vi "Main.vi"() -> ()   [LabVIEW 2021]
uses:
  Controls/Base_Station_Emulator.ctl
  Controls/Cellular_Technology.ctl
  Enum.ctl
  Controls/TCP_FGV.ctl
panel:
  in  "PPCH NB":string(combo)="6"
  in  "UL fre":i64=-95000000
  in  "DL fre":u64=2655000000
  in  "Eutra Bands 4G":string(combo)="3"
  in  "Add_subscriber":T1={"value"="11111111111111111111111111111111", "Add_Subscriber"="//add_subscriber", "N"=1, "imsi"="10.2.0.1", "phone_no"=0, "key_value"="8baf473f2f8fd09487cccbd7097c6862", "op/opc_value"="opc", "mnc-length"=""} {"phone_no" min=0 max=2; "N" min=1 max=2}
  in  "Hardware input":T2(ring)
  in  "Tab":enum32{"2G", "4G", "5G"}(tab)
  in  "cell":T3(ring)
  in  "Phy":T4(ring)
  in  "gprs":T5(ring)
  in  "Config2G":enum16{"Hardware", "cell", "phy", "gprs"}(ring)
  in  "UL POWER":i32=-13
  in  "dl power":i32=-13
  in  "CELL":T6(ring)
  in  "PHY":T7(ring)
  in  "RRC":T8(ring)
  in  "Config4G":enum16{"hardware", "cell", "phy", "rrc"}(ring)
  in  "dl power 2":i32=-13
  in  "UL POWER 2":i32=-13
  in  "Delete_Subscriber":string="//Delete_subscriber"
  in  "Set sim Config":bool
  in  "Cellular Technology":T9
  in  "Base Station":T10
  in  "Enter":bool
  in  "Stop":bool
  in  "stop emulator":bool
  in  "Start":bool
  out "error out":errorcluster
  in  "error in (no error)":errorcluster
  # "2655000000"
  # "-95000000"
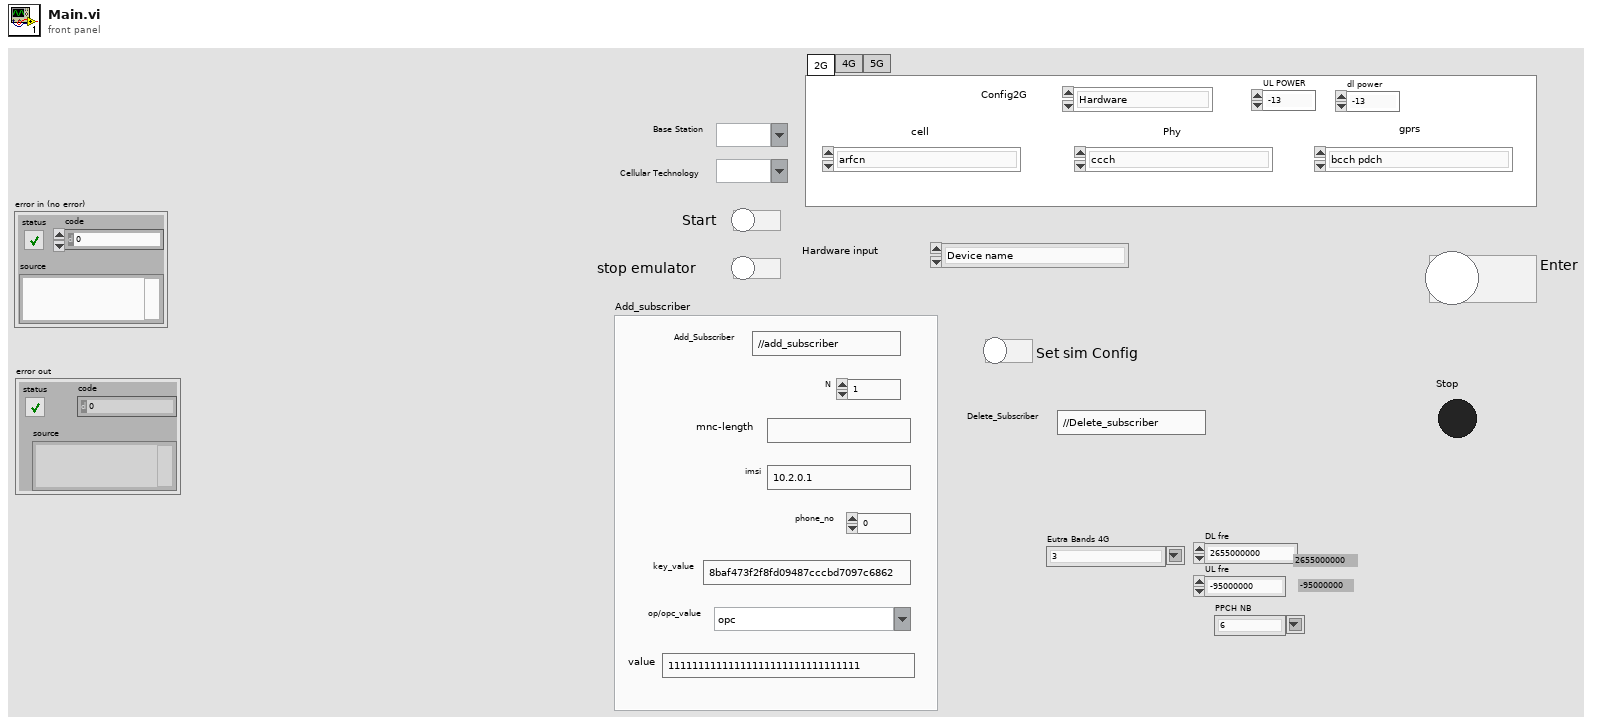
[diagram p1: front panel]
types:
  T1 = cluster{"value":string, "Add_Subscriber":string, "N":i32, "imsi":string, "phone_no":i32, "key_value":string, "op/opc_value":string, "mnc-length":string}
  T2 = enum16{"Device name", "serial name", "dl power", "dl antenna", "ul ref power", "ul antenna"}
  T3 = enum16{"arfcn", "call enables", "cell barred access", "early classmark sending", "fre format", "gprs enabled", "location aea code", "loop back enabled", "mcc", "mnc", "power offset", "si type", "sms enabled"}
  T4 = enum16{"ccch", "add reselect", "attach detach", "block for acs", "cell reselect", "dtx", "hal rate", "min received sig", "multiframe forpg", "pow con indi", "pow contro level", "Rach access control access", "rach call", "RAch maxi retranmission", "rach transmission slots", "radio link timout", "t3212"}
  T5 = enum16{"bcch pdch", "gprs parameter alpha", "access burst", "nack countdown", "network control", "priority access", "rac", "t3168", "t3192"}
  T6 = enum16{"Carrier BW", "DL Frequency", "Duplex Mode", "Eutra operating band", "Measurement report", "MNC length", "MCC", "MNC", "network name", "Physical Cell ID", "Tracking area code", "Transmission Mode", "UL frequency"}
  T7 = enum16{"BCCH modi Coeff", "pbch Repetition", "pcch Narrowband", "pcch pg cycle", "pdsch power boost", "pdsch Ref power", "phich duration", "phish resource", "prach config index", "prach contention resolution", "prach initial received target", "prach maximum transmission", "prach ramping step size", "prach response window", "prach root sequence", "pussh an occassions", "pucch cqi num of RB", "pucch cs antenna", "pucch delta shift", "pucch harq max", "pucch power offset", "pusch alpha", "pusch dmrs enable", "pusch power offset", "srs enable"}
  T8 = enum16{"rlc maxi retransmission", "rlc poll byte", "rlc poll pdu", "rlc timer poll retransmit", "rlc timer reordering", "rlc timer status prohibit"}
  T9 = typedef "Cellular_Technology.ctl" = string
  T10 = typedef "Base_Station_Emulator.ctl" = string
  T11 = typedef "Enum.ctl" = enum16{"Init", "poll", "Start", "Stop", "Config", "Set sim", "Config-4G", "Config-5G"}
  T12 = typedef "TCP_FGV.ctl" = enum16{"Open", "Read", "Write", "Close"}
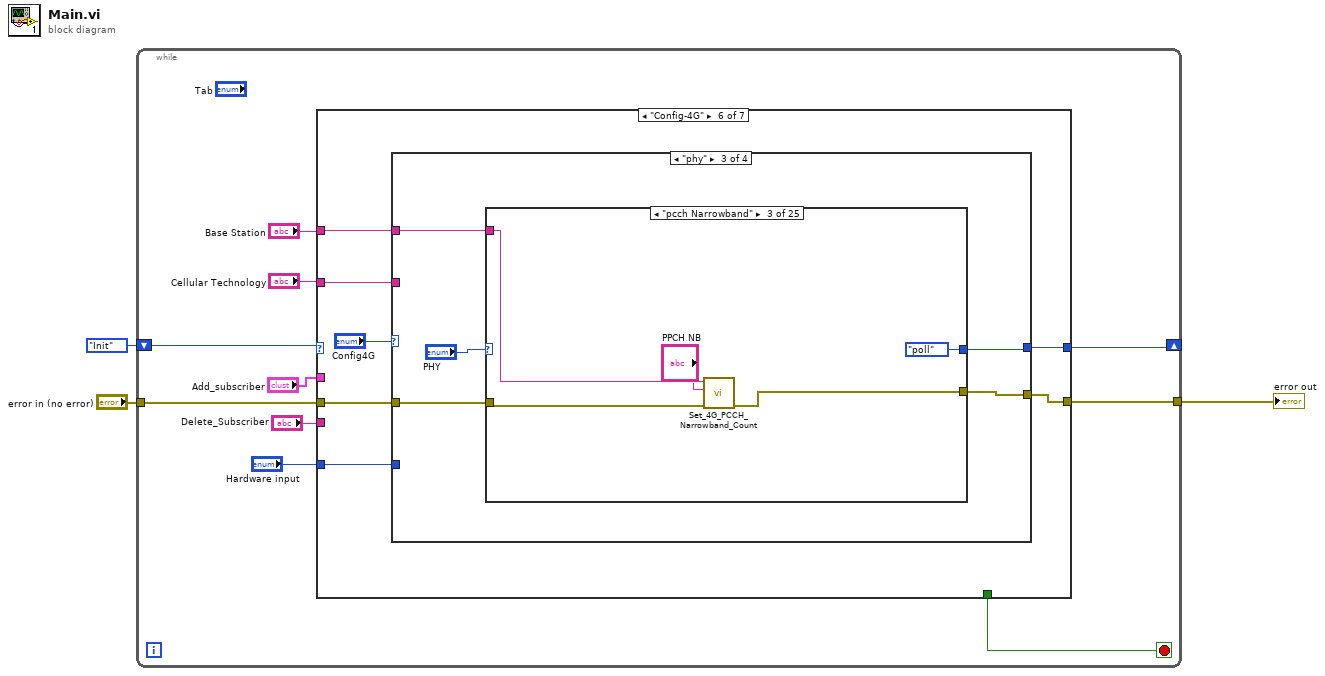
[diagram p0: block diagram]
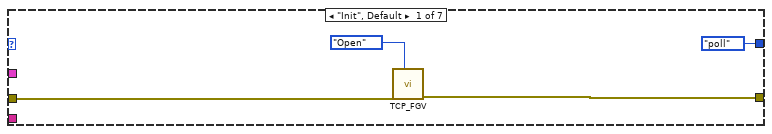
[diagram p2: hidden frame]
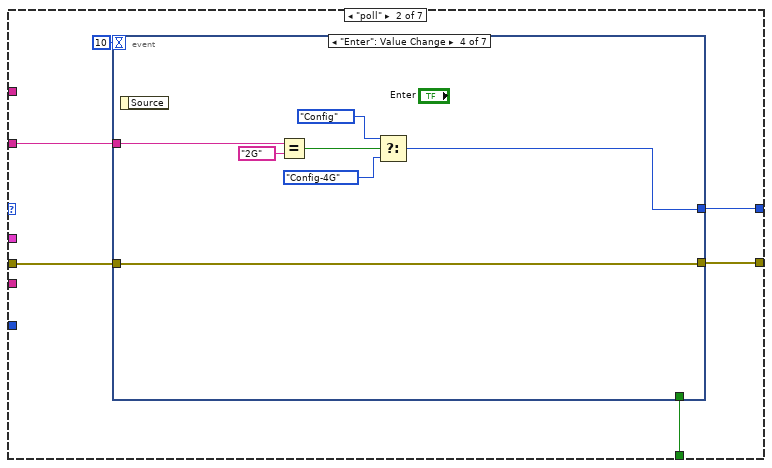
[diagram p3: hidden frame]
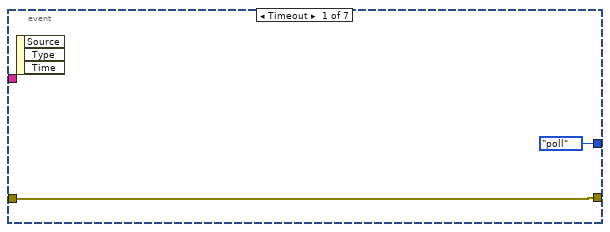
[diagram p4: hidden frame]
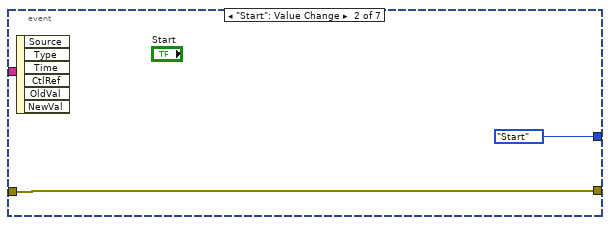
[diagram p5: hidden frame]
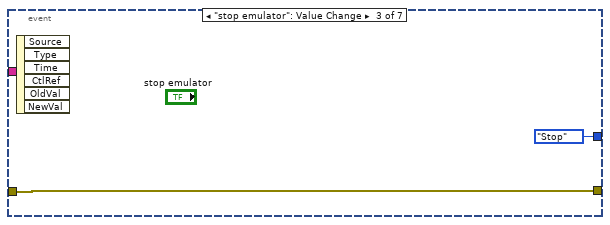
[diagram p6: hidden frame]
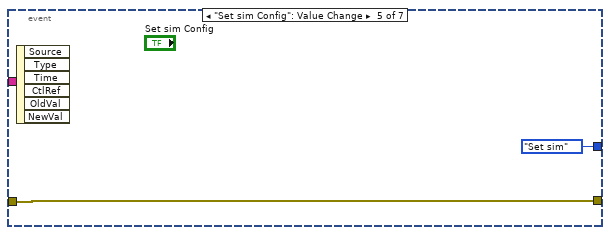
[diagram p7: hidden frame]
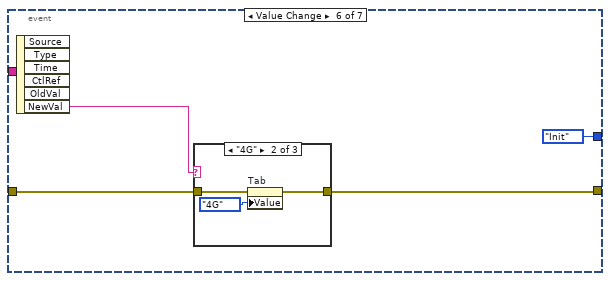
[diagram p8: hidden frame]
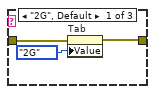
[diagram p9: hidden frame]
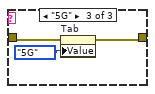
[diagram p10: hidden frame]
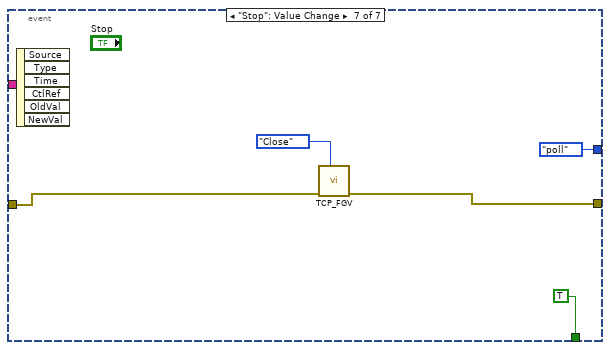
[diagram p11: hidden frame]
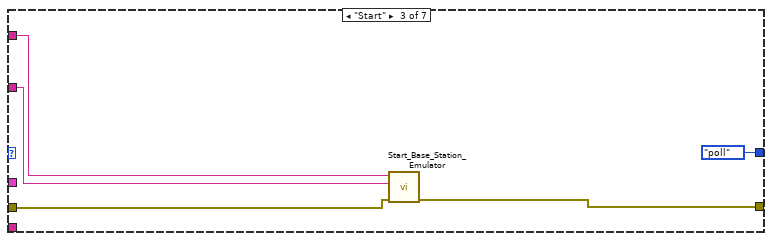
[diagram p12: hidden frame]
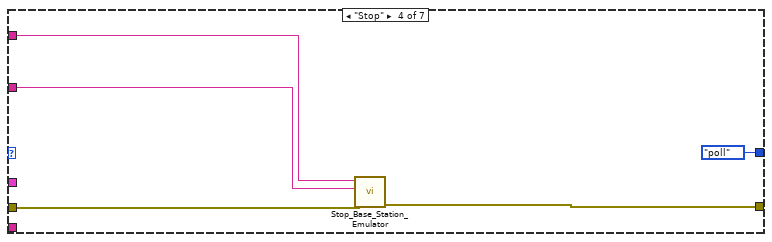
[diagram p13: hidden frame]
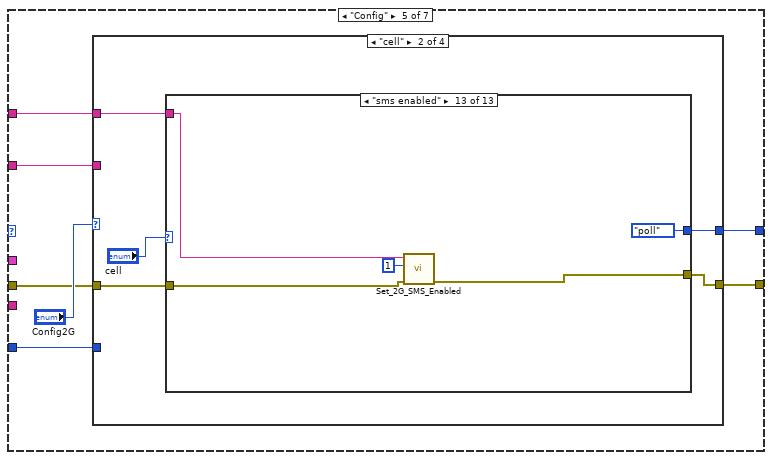
[diagram p14: hidden frame]
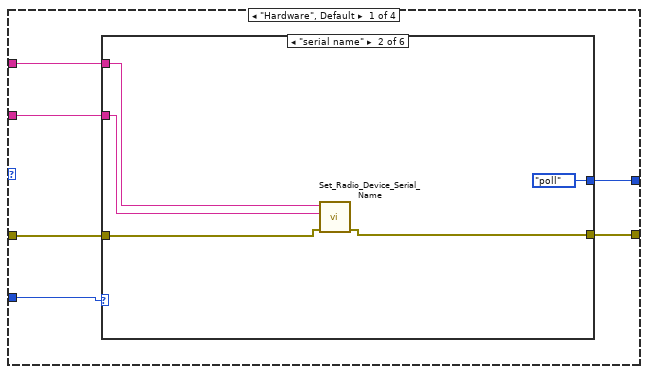
[diagram p15: hidden frame]
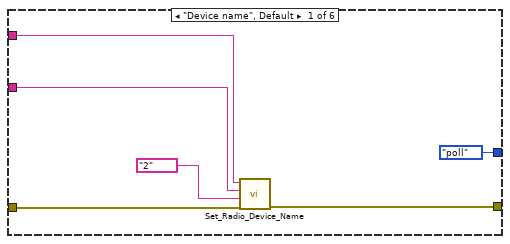
[diagram p16: hidden frame]
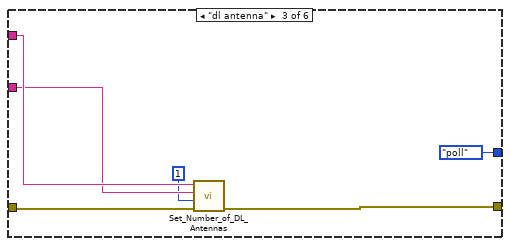
[diagram p17: hidden frame]
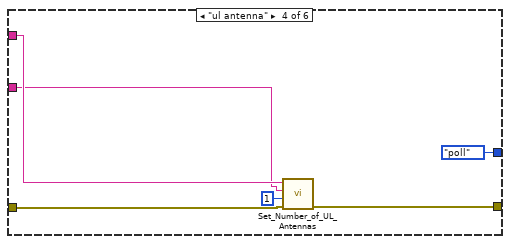
[diagram p18: hidden frame]
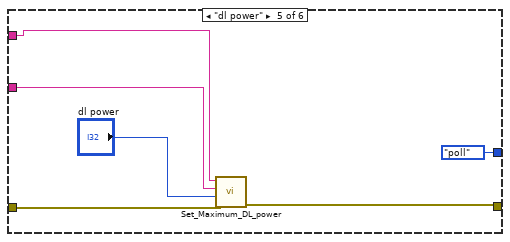
[diagram p19: hidden frame]
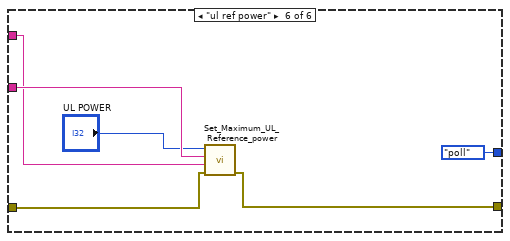
[diagram p20: hidden frame]
diagram:
  n1 = while {
    shift-right: [w12] -> _
    shift-left: Enum."Init" -> [w13]
    tunnel: "error in (no error)" -> [w11]
    tunnel: [w10] -> w1
    stop <- w9 stop-if-true
    n2 = case shown="\"Config-4G\"" w13 {
      tunnel: [Enum."poll" w22 Enum."poll" Enum."poll" w68 w326 w604] -> w12
      tunnel: w11 -> [w16 w21 w61 w66 w72 w330 w608]
      tunnel: [w15 w20 w60 w65 w69 w327 w607] -> w10
      tunnel: "Base Station" -> [_ _ w58 w63 w71 w329 _]
      tunnel: "Cellular Technology" -> [_ w18 w57 w62 w70 w328 _]
      tunnel: "Delete_Subscriber" -> [_ _ _ _ _ _ w606]
      tunnel: [_ w19 _ _ _ _ _] -> w9
      tunnel: "Add_subscriber" -> [_ _ _ _ _ _ w605]
      tunnel: "Hardware input" -> [_ _ _ _ w67 w325 _]
      frame "Init", Default {
        n3 = call "TCP_FGV.vi"("error in (no error)"=w16, "Operation"=TCP_FGV."Open") -> ("error out"=w15:errorcluster)  [unwired: 7 in, 1 out]
      }
      frame "poll" {
        n4 = event shown="[3] \"Enter\": Value Change" {
          selector: _ -> [_ _ _ _ _ _ _]
          dyn-events: _ -> [_ _ _ _ _ _ _]
          timeout: 10 -> [_ _ _ _ _ _ _]
          tunnel: [Enum."poll" Enum."Start" Enum."Stop" w31 Enum."Set sim" Enum."Init" Enum."poll"] -> w22
          tunnel: w21 -> [w24 w26 w28 w36 w38 w41 w54]
          tunnel: [w24 w26 w28 w36 w38 w42 w53] -> w20
          tunnel: [_ _ _ _ _ _ TRUE] -> w19
          tunnel: w18 -> [_ _ _ w35 _ _ _]
          event Timeout {
            n5 = event-data() -> ()  [unwired: 1 in, 3 out]
          }
          event "Start": Value Change {
            n6 = event-data() -> ()  [unwired: 1 in, 6 out]
          }
          event "stop emulator": Value Change {
            n7 = event-data() -> ()  [unwired: 1 in, 6 out]
          }
          event "Enter": Value Change {
            n8 = event-data() -> ()  [unwired: 1 in, 1 out]
            n9 = Equal?(x=w35, y=T9 "2G") -> (x = y?=w33:bool)
            n10 = Select(t=Enum."Config", s=w33, f=Enum."Config-4G") -> (s? t:f=w31:T11)
          }
          event "Set sim Config": Value Change {
            n11 = event-data() -> ()  [unwired: 1 in, 6 out]
          }
          event Value Change {
            n12 = event-data() -> ("NewVal"=w40:T9)  [unwired: 1 in, 5 out]
            n13 = case shown="\"4G\"" w40 {
              tunnel: [w44 w48 w51] -> w42
              tunnel: w41 -> [w45 w47 w50]
              frame "2G", Default {
                n14 = property on="Tab" class="TabCtl (strict)"(error in=w45, "Value"=enum32{"2G", "4G", "5G"}."2G" ("Tab")) -> (error out=w44:errorcluster)  [unwired: 1 in, 1 out]
              }
              frame "4G" {
                n15 = property on="Tab" class="TabCtl (strict)"(error in=w47, "Value"=enum32{"2G", "4G", "5G"}."4G" ("Tab")) -> (error out=w48:errorcluster)  [unwired: 1 in, 1 out]
              }
              frame "5G" {
                n16 = property on="Tab" class="TabCtl (strict)"(error in=w50, "Value"=enum32{"2G", "4G", "5G"}."5G" ("Tab")) -> (error out=w51:errorcluster)  [unwired: 1 in, 1 out]
              }
            }
          }
          event "Stop": Value Change {
            n17 = event-data() -> ()  [unwired: 1 in, 6 out]
            n18 = call "TCP_FGV.vi"("error in (no error)"=w54, "Operation"=TCP_FGV."Close") -> ("error out"=w53:errorcluster)  [unwired: 7 in, 1 out]
          }
        }
      }
      frame "Start" {
        n19 = call "Start_Base_Station_Emulator.vi"("error in (no error)"=w61, "Cellular Technology"=w57, "Base Station"=w58) -> ("error out"=w60:errorcluster)  [unwired: 7 in, 1 out]
      }
      frame "Stop" {
        n20 = call "Stop_Base_Station_Emulator.vi"("error in (no error)"=w66, "Cellular Technology"=w62, "Base Station"=w63) -> ("error out"=w65:errorcluster)  [unwired: 7 in, 1 out]
      }
      frame "Config" {
        n21 = case shown="\"cell\"" "Config2G" {
          tunnel: w72 -> [w79 w117 w188 w277]
          tunnel: w71 -> [w78 w116 w185 w275]
          tunnel: w70 -> [w77 _ _ _]
          tunnel: [w76 w115 w187 w276] -> w69
          tunnel: [w75 w118 w186 w279] -> w68
          tunnel: w67 -> [w74 _ _ _]
          frame "Hardware", Default {
            n22 = case shown="\"serial name\"" w74 {
              tunnel: w79 -> [w85 w90 w94 w102 w108 w112]
              tunnel: [w84 w89 w93 w101 w107 w111] -> w76
              tunnel: w78 -> [w83 w88 w96 w100 w105 w113]
              tunnel: w77 -> [w82 w87 w95 w99 w104 w114]
              tunnel: [Enum."poll" Enum."poll" Enum."poll" Enum."poll" Enum."poll" Enum."poll"] -> w75
              frame "Device name", Default {
                n23 = call "Set_Radio_Device_Name.vi"("error in (no error)"=w85, "value"="2", "Cellular Technology"=w82, "Base Station"=w83) -> ("error out"=w84:errorcluster)  [unwired: 6 in, 1 out]
              }
              frame "serial name" {
                n24 = call "Set_Radio_Device_Serial_Name.vi"("error in (no error)"=w90, "Cellular Technology"=w87, "Base Station"=w88) -> ("error out"=w89:errorcluster)  [unwired: 7 in, 1 out]
              }
              frame "dl antenna" {
                n25 = call "Set_Number_of_DL_Antennas.vi"("error in (no error)"=w94, "No of DL antennas Value"=1, "Cellular Technology"=w95, "Base Station"=w96) -> ("error out"=w93:errorcluster)  [unwired: 6 in, 1 out]
              }
              frame "ul antenna" {
                n26 = call "Set_Number_of_UL_Antennas.vi"("error in (no error)"=w102, "No of UL antennas Value"=1, "Cellular Technology"=w99, "Base Station"=w100) -> ("error out"=w101:errorcluster)  [unwired: 6 in, 1 out]
              }
              frame "dl power" {
                n27 = call "Set_Maximum_DL_power.vi"("error in (no error)"=w108, "No of DL antennas Value"="dl power", "Cellular Technology"=w104, "Base Station"=w105) -> ("error out"=w107:errorcluster)  [unwired: 6 in, 1 out]
              }
              frame "ul ref power" {
                n28 = call "Set_Maximum_UL_Reference_power.vi"("error in (no error)"=w112, "Base Station"=w113, "Cellular Technology"=w114, "No of DL antennas Value"="UL POWER") -> ("error out"=w111:errorcluster)  [unwired: 6 in, 1 out]
              }
            }
          }
          frame "cell" {
            n29 = case shown="\"sms enabled\"" "cell" {
              tunnel: [Enum."poll" Enum."poll" Enum."poll" Enum."poll" Enum."poll" Enum."poll" Enum."poll" Enum."poll" Enum."poll" Enum."poll" Enum."poll" Enum."poll" Enum."poll"] -> w118
              tunnel: w117 -> [w123 w129 w134 w138 w144 w149 w154 w158 w164 w169 w174 w179 w184]
              tunnel: w116 -> [w122 w127 w131 w136 w142 w147 w151 w156 w161 w166 w171 w177 w181]
              tunnel: [w120 w128 w133 w137 w143 w148 w153 w157 w163 w168 w173 w178 w183] -> w115
              frame "arfcn", Default {
                n30 = call "Set_2G_ARFCN.vi"("error in (no error)"=w123, "value"=51, "Base Station"=w122) -> ("error out"=w120:errorcluster)  [unwired: 7 in, 1 out]
              }
              frame "call enables" {
                n31 = call "Set_2G_Call_Enabled.vi"("error in (no error)"=w129, "value"=0, "Base Station"=w127) -> ("error out"=w128:errorcluster)  [unwired: 7 in, 1 out]
              }
              frame "cell barred access" {
                n32 = call "Set_2G_Cell_Barred_Access.vi"("error in (no error)"=w134, "value"=0, "Base Station"=w131) -> ("error out"=w133:errorcluster)  [unwired: 7 in, 1 out]
              }
              frame "early classmark sending" {
                n33 = call "Set_2G_Early_Classmark_Sending_Control.vi"("error in (no error)"=w138, "value"=0, "Base Station"=w136) -> ("error out"=w137:errorcluster)  [unwired: 7 in, 1 out]
              }
              frame "fre format" {
                n34 = call "Set_2G_Frequency_Format_ID.vi"("error in (no error)"=w144, "value"=71, "Base Station"=w142) -> ("error out"=w143:errorcluster)  [unwired: 7 in, 1 out]
              }
              frame "gprs enabled" {
                n35 = call "Set_2G_Location_Area_Code.vi"("error in (no error)"=w149, "value"=0, "Base Station"=w147) -> ("error out"=w148:errorcluster)  [unwired: 7 in, 1 out]
              }
              frame "location aea code" {
                n36 = call "Set_2G_Location_Area_Code.vi"("error in (no error)"=w154, "value"=0, "Base Station"=w151) -> ("error out"=w153:errorcluster)  [unwired: 7 in, 1 out]
              }
              frame "loop back enabled" {
                n37 = call "Set_2G_Loop_Back_Enabled.vi"("error in (no error)"=w158, "value"=0, "Base Station"=w156) -> ("error out"=w157:errorcluster)  [unwired: 7 in, 1 out]
              }
              frame "mcc" {
                n38 = call "Set_2G_Mobile_Country_Code.vi"("error in (no error)"=w164, "value"=0, "Base Station"=w161) -> ("error out"=w163:errorcluster)  [unwired: 7 in, 1 out]
              }
              frame "mnc" {
                n39 = call "Set_2G_Mobile_Network_Code.vi"("error in (no error)"=w169, "value"=0, "Base Station"=w166) -> ("error out"=w168:errorcluster)  [unwired: 7 in, 1 out]
              }
              frame "power offset" {
                n40 = call "Set_2G_power_offset_indicator.vi"("error in (no error)"=w174, "value"=0, "Base Station"=w171) -> ("error out"=w173:errorcluster)  [unwired: 7 in, 1 out]
              }
              frame "si type" {
                n41 = call "Set_2G_si_type2_ter_indicator.vi"("error in (no error)"=w179, "value"=0, "Base Station"=w177) -> ("error out"=w178:errorcluster)  [unwired: 7 in, 1 out]
              }
              frame "sms enabled" {
                n42 = call "Set_2G_SMS_Enabled.vi"("error in (no error)"=w184, "value"=1, "Base Station"=w181) -> ("error out"=w183:errorcluster)  [unwired: 7 in, 1 out]
              }
            }
          }
          frame "phy" {
            n43 = case shown="\"hal rate\"" "Phy" {
              tunnel: w188 -> [w194 w199 w204 w209 w214 w218 w224 w229 w234 w239 w244 w249 w254 w259 w264 w269 w274]
              tunnel: [w193 w198 w203 w208 w213 w217 w223 w228 w233 w238 w243 w248 w253 w257 w263 w268 w273] -> w187
              tunnel: [Enum."poll" Enum."poll" Enum."poll" Enum."poll" Enum."poll" Enum."poll" Enum."poll" Enum."poll" Enum."poll" Enum."poll" Enum."poll" Enum."poll" Enum."poll" Enum."poll" Enum."poll" Enum."poll" Enum."poll"] -> w186
              tunnel: w185 -> [w191 w197 w201 w206 w211 w216 w221 w226 w231 w236 w241 w247 w251 w258 w261 w266 w271]
              frame "ccch", Default {
                n44 = call "Set 2G CCCH Combination.vi"("error in (no error)"=w194, "value"=1, "Base Station"=w191) -> ("error out"=w193:errorcluster)  [unwired: 7 in, 1 out]
              }
              frame "add reselect" {
                n45 = call "Set_2G_Add_Reselect_Indicator.vi"("error in (no error)"=w199, "value"=0, "Base Station"=w197) -> ("error out"=w198:errorcluster)  [unwired: 7 in, 1 out]
              }
              frame "attach detach" {
                n46 = call "Set_2G_Attach_Detach_Allowed.vi"("error in (no error)"=w204, "value"=0, "Base Station"=w201) -> ("error out"=w203:errorcluster)  [unwired: 7 in, 1 out]
              }
              frame "block for acs" {
                n47 = call "Set_2G_Block_For_Access_Grant.vi"("error in (no error)"=w209, "value"=3, "Base Station"=w206) -> ("error out"=w208:errorcluster)  [unwired: 7 in, 1 out]
              }
              frame "cell reselect" {
                n48 = call "Set_2G_Cell_Reselect_Hysteresis.vi"("error in (no error)"=w214, "value"=2, "Base Station"=w211) -> ("error out"=w213:errorcluster)  [unwired: 7 in, 1 out]
              }
              frame "dtx" {
                n49 = call "Set_2G_DTX_Indicator.vi"("error in (no error)"=w218, "value"=2, "Base Station"=w216) -> ("error out"=w217:errorcluster)  [unwired: 7 in, 1 out]
              }
              frame "hal rate" {
                n50 = call "Set_2G_Half_Rate_Support.vi"("error in (no error)"=w224, "value"=0, "Base Station"=w221) -> ("error out"=w223:errorcluster)  [unwired: 7 in, 1 out]
              }
              frame "min received sig" {
                n51 = call "Set_2G_Minimum_Received_Signal_Level.vi"("error in (no error)"=w229, "value"=16, "Base Station"=w226) -> ("error out"=w228:errorcluster)  [unwired: 7 in, 1 out]
              }
              frame "multiframe forpg" {
                n52 = call "Set_2G_Multiframe_For_Paging.vi"("error in (no error)"=w234, "value"=3, "Base Station"=w231) -> ("error out"=w233:errorcluster)  [unwired: 7 in, 1 out]
              }
              frame "pow con indi" {
                n53 = call "Set_2G_Power_Control_Indicator.vi"("error in (no error)"=w239, "value"=0, "Base Station"=w236) -> ("error out"=w238:errorcluster)  [unwired: 7 in, 1 out]
              }
              frame "pow contro level" {
                n54 = call "Set_2G_Power_Control_Level .vi"("error in (no error)"=w244, "value"=31, "Base Station"=w241) -> ("error out"=w243:errorcluster)  [unwired: 7 in, 1 out]
              }
              frame "Rach access control access" {
                n55 = call "Set_2G_RACH_Access_Control_Class.vi"("error in (no error)"=w249, "value"=0, "Base Station"=w247) -> ("error out"=w248:errorcluster)  [unwired: 7 in, 1 out]
              }
              frame "rach call" {
                n56 = call "Set_2G_RACH_Call_Reestablishment.vi"("error in (no error)"=w254, "value"=1, "Base Station"=w251) -> ("error out"=w253:errorcluster)  [unwired: 7 in, 1 out]
              }
              frame "RAch maxi retranmission" {
                n57 = call "Set_2G_RACH_Maximum_Retransmission.vi"("error in (no error)"=w259, "value"=1, "Base Station"=w258) -> ("error out"=w257:errorcluster)  [unwired: 7 in, 1 out]
              }
              frame "rach transmission slots" {
                n58 = call "Set_2G_RACH_Transmission_Slots.vi"("error in (no error)"=w264, "value"=14, "Base Station"=w261) -> ("error out"=w263:errorcluster)  [unwired: 7 in, 1 out]
              }
              frame "radio link timout" {
                n59 = call "Set_2G_Radio_Link_Timeout.vi"("error in (no error)"=w269, "value"=1, "Base Station"=w266) -> ("error out"=w268:errorcluster)  [unwired: 7 in, 1 out]
              }
              frame "t3212" {
                n60 = call "Set_2G_t3212.vi"("error in (no error)"=w274, "value"=1, "Base Station"=w271) -> ("error out"=w273:errorcluster)  [unwired: 7 in, 1 out]
              }
            }
          }
          frame "gprs" {
            n61 = case shown="\"network control\"" "gprs" {
              tunnel: [Enum."poll" Enum."poll" Enum."poll" Enum."poll" Enum."poll" Enum."poll" Enum."poll" Enum."poll" Enum."poll"] -> w279
              tunnel: w277 -> [w284 w288 w294 w299 w304 w309 w314 w319 w324]
              tunnel: [w283 w287 w293 w298 w303 w308 w313 w318 w323] -> w276
              tunnel: w275 -> [w281 w286 w291 w296 w301 w306 w311 w316 w321]
              frame "bcch pdch", Default {
                n62 = call "Set_2G_GPRS _BCCH_PDCH_Measurement.vi"("error in (no error)"=w284, "value"=0, "Base Station"=w281) -> ("error out"=w283:errorcluster)  [unwired: 7 in, 1 out]
              }
              frame "gprs parameter alpha" {
                n63 = call "Set_2G_GPRS_Parameter_Alpha.vi"("error in (no error)"=w288, "value"=1, "Base Station"=w286) -> ("error out"=w287:errorcluster)  [unwired: 7 in, 1 out]
              }
              frame "access burst" {
                n64 = call "Set_GPRS_Access_Burst_Type.vi"("error in (no error)"=w294, "value"="TM1", "Base Station"=w291) -> ("error out"=w293:errorcluster)  [unwired: 7 in, 1 out]
              }
              frame "nack countdown" {
                n65 = call "Set_GPRS_NACK_Countdown.vi"("error in (no error)"=w299, "value"=8, "Base Station"=w296) -> ("error out"=w298:errorcluster)  [unwired: 7 in, 1 out]
              }
              frame "network control" {
                n66 = call "Set_GPRS_Network_Control_Order.vi"("error in (no error)"=w304, "value"=0, "Base Station"=w301) -> ("error out"=w303:errorcluster)  [unwired: 7 in, 1 out]
              }
              frame "priority access" {
                n67 = call "Set_GPRS_Priority_Access_THR.vi"("error in (no error)"=w309, "value"=6, "Base Station"=w306) -> ("error out"=w308:errorcluster)  [unwired: 7 in, 1 out]
              }
              frame "rac" {
                n68 = call "Set_GPRS_RAC.vi"("error in (no error)"=w314, "value"="128", "Base Station"=w311) -> ("error out"=w313:errorcluster)  [unwired: 7 in, 1 out]
              }
              frame "t3168" {
                n69 = call "Set_GPRS_t3168.vi"("error in (no error)"=w319, "value"=0, "Base Station"=w316) -> ("error out"=w318:errorcluster)  [unwired: 7 in, 1 out]
              }
              frame "t3192" {
                n70 = call "Set_GPRS_t3192.vi"("error in (no error)"=w324, "value"=0, "Base Station"=w321) -> ("error out"=w323:errorcluster)  [unwired: 7 in, 1 out]
              }
            }
          }
        }
      }
      frame "Config-4G" {
        n71 = case shown="\"phy\"" "Config4G" {
          tunnel: w330 -> [w335 w375 w442 w571]
          tunnel: w329 -> [w333 w374 w439 w569]
          tunnel: w328 -> [w334 _ _ _]
          tunnel: [w336 w373 w441 w570] -> w327
          tunnel: [w337 w376 w440 w573] -> w326
          tunnel: w325 -> [w332 _ _ _]
          frame "hardware" {
            n72 = case shown="\"Device name\", Default" w332 {
              tunnel: w335 -> [w343 w348 w352 w360 w366 w370]
              tunnel: [w342 w347 w351 w359 w365 w369] -> w336
              tunnel: w333 -> [w341 w346 w354 w358 w363 w371]
              tunnel: w334 -> [w340 w345 w353 w357 w362 w372]
              tunnel: [Enum."poll" Enum."poll" Enum."poll" Enum."poll" Enum."poll" Enum."poll"] -> w337
              frame "Device name", Default {
                n73 = call "Set_Radio_Device_Name.vi"("error in (no error)"=w343, "value"="0", "Cellular Technology"=w340, "Base Station"=w341) -> ("error out"=w342:errorcluster)  [unwired: 6 in, 1 out]
              }
              frame "serial name" {
                n74 = call "Set_Radio_Device_Serial_Name.vi"("error in (no error)"=w348, "Cellular Technology"=w345, "Base Station"=w346) -> ("error out"=w347:errorcluster)  [unwired: 7 in, 1 out]
              }
              frame "dl antenna" {
                n75 = call "Set_Number_of_DL_Antennas.vi"("error in (no error)"=w352, "No of DL antennas Value"=1, "Cellular Technology"=w353, "Base Station"=w354) -> ("error out"=w351:errorcluster)  [unwired: 6 in, 1 out]
              }
              frame "ul antenna" {
                n76 = call "Set_Number_of_UL_Antennas.vi"("error in (no error)"=w360, "No of UL antennas Value"=1, "Cellular Technology"=w357, "Base Station"=w358) -> ("error out"=w359:errorcluster)  [unwired: 6 in, 1 out]
              }
              frame "dl power" {
                n77 = call "Set_Maximum_DL_power.vi"("error in (no error)"=w366, "No of DL antennas Value"="dl power 2", "Cellular Technology"=w362, "Base Station"=w363) -> ("error out"=w365:errorcluster)  [unwired: 6 in, 1 out]
              }
              frame "ul ref power" {
                n78 = call "Set_Maximum_UL_Reference_power.vi"("error in (no error)"=w370, "Base Station"=w371, "Cellular Technology"=w372, "No of DL antennas Value"="UL POWER 2") -> ("error out"=w369:errorcluster)  [unwired: 6 in, 1 out]
              }
            }
          }
          frame "cell" {
            n79 = case shown="\"UL frequency\"" "CELL" {
              tunnel: [Enum."poll" Enum."poll" Enum."poll" Enum."poll" Enum."poll" Enum."poll" Enum."poll" Enum."poll" Enum."poll" Enum."poll" Enum."poll" Enum."poll" Enum."poll"] -> w376
              tunnel: w375 -> [w381 w386 w391 w396 w400 w405 w409 w413 w417 w422 w427 w432 w437]
              tunnel: w374 -> [w380 w385 w390 w395 w399 w404 w408 w412 _ w421 w426 w431 w436]
              tunnel: [w379 w384 w389 w394 w398 w403 w407 w411 w416 w420 w425 w430 w435] -> w373
              frame "Carrier BW" {
                n80 = call "Set_4G_Carrier_Bandwidth.vi"("error in (no error)"=w381, "value"="10", "Base Station"=w380) -> ("error out"=w379:errorcluster)  [unwired: 7 in, 1 out]
              }
              frame "DL Frequency" {
                (unwired) u64 2655000000 ("value")
                n81 = call "Set_4G_DL_Frequency.vi"("error in (no error)"=w386, "value"="DL fre", "Base Station"=w385) -> ("error out"=w384:errorcluster)  [unwired: 7 in, 1 out]
              }
              frame "Duplex Mode" {
                n82 = call "Set_4G_Duplex_Mode.vi"("error in (no error)"=w391, "value"="0", "Base Station"=w390) -> ("error out"=w389:errorcluster)  [unwired: 7 in, 1 out]
              }
              frame "Eutra operating band" {
                n83 = call "Set_4G_EUTRA_Operating_Band.vi"("error in (no error)"=w396, "value"="Eutra Bands 4G", "Base Station"=w395) -> ("error out"=w394:errorcluster)  [unwired: 7 in, 1 out]
              }
              frame "Measurement report" {
                n84 = call "Set_4G_Measurement_Report.vi"("error in (no error)"=w400, "Base Station"=w399) -> ("error out"=w398:errorcluster)  [unwired: 8 in, 1 out]
              }
              frame "MNC length" {
                n85 = call "Set_4G_MNC_length.vi"("error in (no error)"=w405, "value"=2, "Base Station"=w404) -> ("error out"=w403:errorcluster)  [unwired: 7 in, 1 out]
              }
              frame "MCC" {
                n86 = call "Set_4G_Mobile_Country_Code.vi"("error in (no error)"=w409, "Base Station"=w408) -> ("error out"=w407:errorcluster)  [unwired: 8 in, 1 out]
              }
              frame "MNC" {
                n87 = call "Set_4G_Mobile_Network_Code.vi"("error in (no error)"=w413, "Base Station"=w412) -> ("error out"=w411:errorcluster)  [unwired: 8 in, 1 out]
              }
              frame "network name" {
                n88 = call "Set_4G_Network_Name.vi"("error in (no error)"=w417, "value"="MaxEye") -> ("error out"=w416:errorcluster)  [unwired: 8 in, 1 out]
              }
              frame "Physical Cell ID" {
                n89 = call "Set_4G_Physical_Cell_ID.vi"("error in (no error)"=w422, "value"=0, "Base Station"=w421) -> ("error out"=w420:errorcluster)  [unwired: 7 in, 1 out]
              }
              frame "Tracking area code" {
                n90 = call "Set_4G_Tracking_Area_Code.vi"("error in (no error)"=w427, "value"=1, "Base Station"=w426) -> ("error out"=w425:errorcluster)  [unwired: 7 in, 1 out]
              }
              frame "Transmission Mode" {
                n91 = call "Set_4G_Transmission_Mode.vi"("error in (no error)"=w432, "value"="TM1", "Base Station"=w431) -> ("error out"=w430:errorcluster)  [unwired: 7 in, 1 out]
              }
              frame "UL frequency" {
                (unwired) i64 -95000000 ("value")
                n92 = call "Set_4G_UL_Frequency.vi"("error in (no error)"=w437, "value"="UL fre", "Base Station"=w436) -> ("error out"=w435:errorcluster)  [unwired: 7 in, 1 out]
              }
            }
          }
          frame "phy" {
            n93 = case shown="\"pcch Narrowband\"" "PHY" {
              tunnel: w442 -> [w448 w453 w458 w463 w468 w472 w478 w483 w488 w493 w498 w503 w508 w513 w518 w523 w528 w533 w538 w543 w548 w553 w558 w563 w568]
              tunnel: [w447 w452 w457 w462 w467 w471 w477 w482 w487 w492 w497 w502 w506 w512 w517 w522 w527 w532 w537 w542 w547 w552 w557 w562 w567] -> w441
              tunnel: [Enum."poll" Enum."poll" Enum."poll" Enum."poll" Enum."poll" Enum."poll" Enum."poll" Enum."poll" Enum."poll" Enum."poll" Enum."poll" Enum."poll" Enum."poll" Enum."poll" Enum."poll" Enum."poll" Enum."poll" Enum."poll" Enum."poll" Enum."poll" Enum."poll" Enum."poll" Enum."poll" Enum."poll" Enum."poll"] -> w440
              tunnel: w439 -> [w445 w451 w455 w460 w465 w470 w475 w480 w485 w490 w496 w500 w507 w510 w515 w520 w525 w530 w535 w540 w545 w550 w555 w560 w565]
              frame "BCCH modi Coeff", Default {
                n94 = call "Set_4G_BCCH_Modification_Coefficient .vi"("error in (no error)"=w448, "value"="2", "Base Station"=w445) -> ("error out"=w447:errorcluster)  [unwired: 7 in, 1 out]
              }
              frame "pbch Repetition" {
                n95 = call "Set_4G_PBCH_Repetition.vi"("error in (no error)"=w453, "value"=0, "Base Station"=w451) -> ("error out"=w452:errorcluster)  [unwired: 7 in, 1 out]
              }
              frame "pcch Narrowband" {
                n96 = call "Set_4G_PCCH_Narrowband_Count.vi"("error in (no error)"=w458, "value"="PPCH NB", "Base Station"=w455) -> ("error out"=w457:errorcluster)  [unwired: 7 in, 1 out]
              }
              frame "pcch pg cycle" {
                n97 = call "Set_4G_PCCH_Paging_Cycle.vi"("error in (no error)"=w463, "value"="256", "Base Station"=w460) -> ("error out"=w462:errorcluster)  [unwired: 7 in, 1 out]
              }
              frame "pdsch power boost" {
                n98 = call "Set_4G_PDSCH_Power_Boost.vi"("error in (no error)"=w468, "value"=0, "Base Station"=w465) -> ("error out"=w467:errorcluster)  [unwired: 7 in, 1 out]
              }
              frame "pdsch Ref power" {
                n99 = call "Set_4G_PDSCH_Reference_Power.vi"("error in (no error)"=w472, "value"=-27, "Base Station"=w470) -> ("error out"=w471:errorcluster)  [unwired: 7 in, 1 out]
              }
              frame "phich duration" {
                n100 = call "Set_4G_PHICH_Duration.vi"("error in (no error)"=w478, "value"=0, "Base Station"=w475) -> ("error out"=w477:errorcluster)  [unwired: 7 in, 1 out]
              }
              frame "phish resource" {
                n101 = call "Set_4G_PHICH_Resource.vi"("error in (no error)"=w483, "value"="1", "Base Station"=w480) -> ("error out"=w482:errorcluster)  [unwired: 7 in, 1 out]
              }
              frame "prach config index" {
                n102 = call "Set_4G_PRACH_Configuration_Index.vi"("error in (no error)"=w488, "value"=0, "Base Station"=w485) -> ("error out"=w487:errorcluster)  [unwired: 7 in, 1 out]
              }
              frame "prach contention resolution" {
                n103 = call "Set_4G_PRACH_Contention_Resolution_Timer.vi"("error in (no error)"=w493, "value"="48", "Base Station"=w490) -> ("error out"=w492:errorcluster)  [unwired: 7 in, 1 out]
              }
              frame "prach initial received target" {
                n104 = call "Set_4G_PRACH_Initial_Received_Target_Power.vi"("error in (no error)"=w498, "value"="-108", "Base Station"=w496) -> ("error out"=w497:errorcluster)  [unwired: 7 in, 1 out]
              }
              frame "prach maximum transmission" {
                n105 = call "Set_4G_PRACH_Maximum_Transmissions.vi"("error in (no error)"=w503, "value"="10", "Base Station"=w500) -> ("error out"=w502:errorcluster)  [unwired: 7 in, 1 out]
              }
              frame "prach ramping step size" {
                n106 = call "Set_4G_PRACH_Ramping_Step_Size.vi"("error in (no error)"=w508, "value"="4", "Base Station"=w507) -> ("error out"=w506:errorcluster)  [unwired: 7 in, 1 out]
              }
              frame "prach response window" {
                n107 = call "Set_4G_PRACH_Response_Window_Size.vi"("error in (no error)"=w513, "value"="10", "Base Station"=w510) -> ("error out"=w512:errorcluster)  [unwired: 7 in, 1 out]
              }
              frame "prach root sequence" {
                n108 = call "Set_4G_PRACH_Root_Sequence_Index.vi"("error in (no error)"=w518, "value"=0, "Base Station"=w515) -> ("error out"=w517:errorcluster)  [unwired: 7 in, 1 out]
              }
              frame "pussh an occassions" {
                n109 = call "Set_4G_PUCCH_An_Occassions.vi"("error in (no error)"=w523, "value"=0, "Base Station"=w520) -> ("error out"=w522:errorcluster)  [unwired: 7 in, 1 out]
              }
              frame "pucch cqi num of RB" {
                n110 = call "Set_4G_PUCCH_CQI_Number_of_RB.vi"("error in (no error)"=w528, "value"=0, "Base Station"=w525) -> ("error out"=w527:errorcluster)  [unwired: 7 in, 1 out]
              }
              frame "pucch cs antenna" {
                n111 = call "Set_4G_PUCCH_CS_Antenna_Ports .vi"("error in (no error)"=w533, "value"=1, "Base Station"=w530) -> ("error out"=w532:errorcluster)  [unwired: 7 in, 1 out]
              }
              frame "pucch delta shift" {
                n112 = call "Set_4G_PUCCH_Delta_Shift.vi"("error in (no error)"=w538, "value"=1, "Base Station"=w535) -> ("error out"=w537:errorcluster)  [unwired: 7 in, 1 out]
              }
              frame "pucch harq max" {
                n113 = call "Set_4G_PUCCH_HARQ_Maximum_Transmissions.vi"("error in (no error)"=w543, "value"=4, "Base Station"=w540) -> ("error out"=w542:errorcluster)  [unwired: 7 in, 1 out]
              }
              frame "pucch power offset" {
                n114 = call "Set_4G_PUCCH_Power_Offset.vi"("error in (no error)"=w548, "value"=-96, "Base Station"=w545) -> ("error out"=w547:errorcluster)  [unwired: 7 in, 1 out]
              }
              frame "pusch alpha" {
                n115 = call "Set_4G_PUSCH_Alpha.vi"("error in (no error)"=w553, "value"="1", "Base Station"=w550) -> ("error out"=w552:errorcluster)  [unwired: 7 in, 1 out]
              }
              frame "pusch dmrs enable" {
                n116 = call "Set_4G_PUSCH_DMRS_Enable.vi"("error in (no error)"=w558, "value"=0, "Base Station"=w555) -> ("error out"=w557:errorcluster)  [unwired: 7 in, 1 out]
              }
              frame "pusch power offset" {
                n117 = call "Set_4G_PUSCH_Power_Offset.vi"("error in (no error)"=w563, "value"=-96, "Base Station"=w560) -> ("error out"=w562:errorcluster)  [unwired: 7 in, 1 out]
              }
              frame "srs enable" {
                n118 = call "Set_4G_SRS_Enable.vi"("error in (no error)"=w568, "value"=0, "Base Station"=w565) -> ("error out"=w567:errorcluster)  [unwired: 7 in, 1 out]
              }
            }
          }
          frame "rrc" {
            n119 = case shown="\"rlc maxi retransmission\", Default" "RRC" {
              tunnel: [Enum."poll" Enum."poll" Enum."poll" Enum."poll" Enum."poll" Enum."poll"] -> w573
              tunnel: w571 -> [w578 w582 w588 w593 w598 w603]
              tunnel: [w577 w581 w587 w592 w597 w602] -> w570
              tunnel: w569 -> [w575 w580 w585 w590 w595 w600]
              frame "rlc maxi retransmission", Default {
                n120 = call "Set_4G_RLC_Maximum_Retransmission_Threshold.vi"("error in (no error)"=w578, "value"="2", "Base Station"=w575) -> ("error out"=w577:errorcluster)  [unwired: 7 in, 1 out]
              }
              frame "rlc poll byte" {
                n121 = call "Set_4G_RLC_Poll_Byte.vi"("error in (no error)"=w582, "value"=25, "Base Station"=w580) -> ("error out"=w581:errorcluster)  [unwired: 7 in, 1 out]
              }
              frame "rlc poll pdu" {
                n122 = call "Set_4G_RLC_poll_PDU.vi"("error in (no error)"=w588, "value"=4, "Base Station"=w585) -> ("error out"=w587:errorcluster)  [unwired: 7 in, 1 out]
              }
              frame "rlc timer poll retransmit" {
                n123 = call "Set_4G_RLC_Timer_Poll_Retransmit.vi"("error in (no error)"=w593, "value"=80, "Base Station"=w590) -> ("error out"=w592:errorcluster)  [unwired: 7 in, 1 out]
              }
              frame "rlc timer reordering" {
                n124 = call "Set_4G_RLC_Timer_Reordering.vi"("error in (no error)"=w598, "value"=35, "Base Station"=w595) -> ("error out"=w597:errorcluster)  [unwired: 7 in, 1 out]
              }
              frame "rlc timer status prohibit" {
                n125 = call "Set_4G_RLC_Timer_Status_Prohibit.vi"("error in (no error)"=w603, "value"=0, "Base Station"=w600) -> ("error out"=w602:errorcluster)  [unwired: 7 in, 1 out]
              }
            }
          }
        }
      }
      frame "Set sim" {
        n126 = case shown="\"Add\", Default" enum16{"Add", "Del", "Add APN"}."Add" {
          tunnel: w608 -> [w613 w618 w620]
          tunnel: [w612 w617 w621] -> w607
          tunnel: w606 -> [_ w616 _]
          tunnel: w605 -> [w611 _ _]
          tunnel: [Enum."poll" Enum."poll" Enum."poll"] -> w604
          frame "Add", Default {
            n127 = call "Add_Subscriber.vi"("error in (no error)"=w613, "Add_subscriber"=w611) -> ("error out"=w612:errorcluster)  [unwired: 8 in, 1 out]
          }
          frame "Del" {
            n128 = call "Delete_Subscriber.vi"("error in (no error)"=w618, "N"=1, "Delete_Subscriber"=w616) -> ("error out"=w617:errorcluster)  [unwired: 7 in, 1 out]
          }
          frame "Add APN" {
            n129 = call "Add_APN.vi"("error in (no error)"=w620) -> ("error out"=w621:errorcluster)  [unwired: 9 in, 1 out]
          }
        }
      }
    }
  }
  "error out" <- w1
